vi "myRIO v1.2 Create Timer IRQ.vi"(4 "Callback VI Reference":T2, 5 "Allow Overwrite Operation? (F)":bool, 7 "Timer ID":u8, 8 "error in (no error)":errorcluster, 9 "Interval (us)":u32, 11 "Resource name":T1 caption="RIO Device") -> (0 "error out":errorcluster)   [LabVIEW 2021]
uses:
  <vilib>/myRIO/Common/Instrument Driver Framework/myRIO v1.0/IRQ/typedefs/Callback VI Ref.ctl
  <vilib>/userDefined/High Color/nirio_resource_hc.ctl
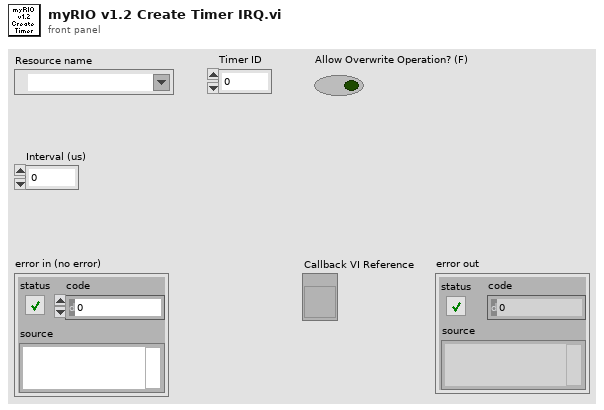
[diagram p1: front panel]
types:
  T1 = typedef "nirio_resource_hc.ctl" = tag
  T2 = typedef "Callback VI Ref.ctl" = refnum<vi>
  T3 = typedef "Generic FPGA Reference.ctl" = refnum<k20>
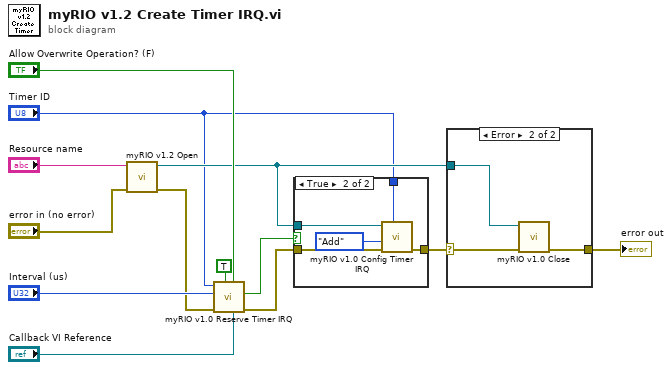
[diagram p0: block diagram]
diagram:
  n1 = call <vilib>:"myRIO v1.2 Open.vi"("error in (no error)"="error in (no error)", "Resource name"="Resource name") -> ("error out"=w4:errorcluster, "myRIO FPGA Ref Out"=w5:T3)  [unwired: 8 in]
  n2 = call <vilib>:"myRIO v1.0 Reserve Timer IRQ.vi"("Callback VI Ref"="Callback VI Reference", "Allow Overwrite?"="Allow Overwrite Operation? (F)", "Reserve?"=TRUE, "error in (no error)"=w4, "Interval(us)"="Interval (us)", "Timer ID"="Timer ID") -> ("error out"=w12:errorcluster, "Succeed?"=w3:bool)  [unwired: 4 in]
  n3 = case shown="True" w3 {
    tunnel: [w14 w19] -> w13
    tunnel: w12 -> [w14 w18]
    tunnel: "Timer ID" -> [_ w17]
    tunnel: w5 -> [_ w16]
    frame False {
    }
    frame True {
      n4 = call <vilib>:"myRIO v1.0 Config Timer IRQ.vi"("Timer ID"=w17, "error in (no error)"=w18, "Action"=enum16{"Add", "Update", "Remove"}."Add", "myRIO FPGA Ref In"=w16) -> ("error out"=w19:errorcluster)  [unwired: 5 in, 2 out]
    }
  }
  n5 = case shown="Error" w13 {
    selector: w13 -> [w20 w23]
    tunnel: w5 -> [_ w21]
    tunnel: [w20 w22] -> w11
    frame No Error {
    }
    frame Error {
      n6 = call <vilib>:"myRIO v1.0 Close.vi"("error in (no error)"=w23, "myRIO FPGA Ref In"=w21) -> ("error out"=w22:errorcluster)  [unwired: 9 in]
    }
  }
  "error out" <- w11
